vi "LED Update Loop.vi"(9 "SPI Clock Rate (Hz)":dbl=7000000.0 format="%#_13g", 11 "update delay (ms)":u32=100) -> ()   [LabVIEW 2014]
uses:
  <vilib>/Rock Robotics/SystemInterfaces/spilib/spi_bus.ctl
  <vilib>/Rock Robotics/WPI/SPI/WPI_SPIMode.ctl
  LED Values.vi
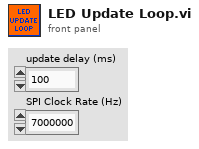
[diagram p1: front panel]
types:
  T1 = typedef "WPI_SPIMode.ctl" = enum16{"Mode 0 (Clk Idle Low,Sample on Leading)", "Mode 1 (Clk Idle Low,Sample on Trailing)", "Mode 2 (Clk Idle High,Sample on Leading)", "Mode 3 (Clk Idle High,Sample on Trailing)"}
  T2 = typedef "spi_bus.ctl" = enum16{"SPI On-Board, CS0", "SPI On-Board, CS1", "SPI On-Board, CS2", "SPI On-Board, CS3", "SPI MXP", "Invalid"}
  T3 = typedef "WPI_SPIDevRef.ctl" = cluster{"DevStatus":errorcluster, "Handle":i32, "Controller":T4, "SPI Bus":T2}
  T4 = typedef "FPGA_TypedefDigitalModule.ctl" = enum16{"Controller 1"}
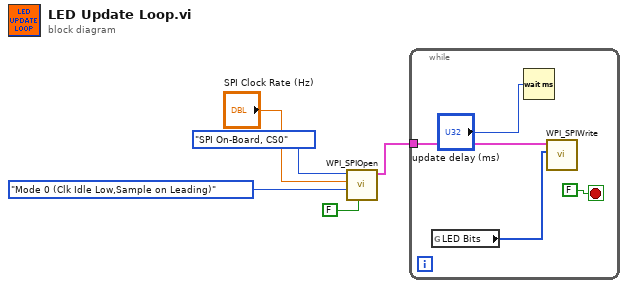
[diagram p0: block diagram]
diagram:
  n1 = call <vilib>:"WPI_SPIOpen.vi"("Chip Select Active High (F)"=FALSE, "Mode (3)"=WPI_SPIMode."Mode 0 (Clk Idle Low,Sample on Leading)", "Clock Rate (Hz)"="SPI Clock Rate (Hz)", "SPI Bus"=spi_bus."SPI On-Board, CS0") -> ("SPIDevRef"=w5:T3)  [unwired: 6 in, 1 out]
  n2 = while {
    tunnel: w5 -> [w9]
    stop <- FALSE stop-if-true
    n3 = global read "LED Values.vi" "LED Bits"() -> (w6:u8[])
    n4 = Wait (ms)(milliseconds to wait="update delay (ms)") -> ()  [unwired: 1 out]
    n5 = call <vilib>:"WPI_SPIWrite.vi"("Data To Send"=w6, "SPIDevRef"=w9) -> ()  [unwired: 7 in, 3 out]
  }
